vi "Control.vi"() -> ()   [LabVIEW 2019]
uses:
  <vilib>/Analysis/NI_AALBase.lvlib
  <vilib>/Analysis/baseanly.llb/Real Dot Product.vi
panel:
  in  "CTR_K":dbl[](array[numeric]) format="%.2f"
  in  "q0":dbl
  in  "q":dbl
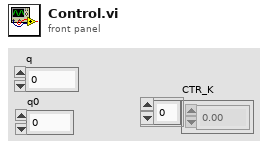
[diagram p1: front panel]
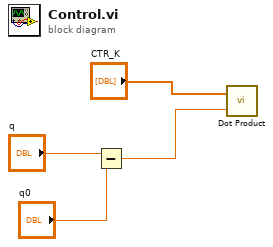
[diagram p0: block diagram]
diagram:
  n1 = Subtract(x="q", y="q0") -> (x-y=w2:dbl)
  n2 = call-poly <vilib>:"Dot Product.vi"("Y Vector"=w2, "X Vector"="CTR_K") -> ()  [unwired: 2 out]
